vi "AD9959controlAS1_B1.vi"(8 "error in (no error)":errorcluster, 9 "Enable Master Stepper":bool, 10 "Array":T2(array[cluster])=[{"Enable ASF?"=FALSE, "Channel Frequency (MHz)"=80.0, "ASF"=0.12, "Enable Frequency Sweep"=FALSE, "Sweep Parameters"={"Start Frequency (MHz)"=80.5, "Stop Frequency (MHz)"=89.25, "Rising Step Size (MHz)"=0.04375, "Falling Step Size (MHz)"=0.0, "Falling Step Interval (ms)"=0.01, "Rising Step Interval (ms)"=1.0}, "Rising/Falling"=FALSE}, {"Enable ASF?"=TRUE, "Channel Frequency (MHz)"=110.0, "ASF"=0.092, "Enable Frequency Sweep"=TRUE, "Sweep Parameters"={"Start Frequency (MHz)"=70.0, "Stop Frequency (MHz)"=130.0, "Rising Step Size (MHz)"=0.015, "Falling Step Size (MHz)"=0.0, "Falling Step Interval (ms)"=0.01, "Rising Step Interval (ms)"=1.0}, "Rising/Falling"=FALSE}, {"Enable ASF?"=FALSE, "Channel Frequency (MHz)"=80.0, "ASF"=0.1, "Enable Frequency Sweep"=FALSE, "Sweep Parameters"={"Start Frequency (MHz)"=80.5, "Stop Frequency (MHz)"=89.25, "Rising Step Size (MHz)"=0.04375, "Falling Step Size (MHz)"=0.0, "Falling Step Interval (ms)"=0.01, "Rising Step Interval (ms)"=1.0}, "Rising/Falling"=FALSE}, {"Enable ASF?"=TRUE, "Channel Frequency (MHz)"=50.0, "ASF"=0.1, "Enable Frequency Sweep"=FALSE, "Sweep Parameters"={"Start Frequency (MHz)"=40.0, "Stop Frequency (MHz)"=115.0, "Rising Step Size (MHz)"=0.0006, "Falling Step Size (MHz)"=0.0, "Falling Step Interval (ms)"=0.01, "Rising Step Interval (ms)"=1.0}, "Rising/Falling"=FALSE}] {"Sweep Parameters"."Rising Step Interval (ms)" min=0.0 max=2.55 step=0.01 format="%.4f"; "Sweep Parameters"."Stop Frequency (MHz)" min=0.0 max=400.0 step=1.0 format="%.6f"; "Sweep Parameters"."Start Frequency (MHz)" min=0.0 max=400.0 step=1.0 format="%.6f"; "Sweep Parameters"."Falling Step Interval (ms)" min=0.0 max=2.55 step=0.01 format="%.2f"; "Sweep Parameters"."Falling Step Size (MHz)" min=0.0 max=400.0 step=0.1 format="%.6f"; "Sweep Parameters"."Rising Step Size (MHz)" min=0.0 max=400.0 step=0.1 format="%.7f"; "ASF" min=0.0 max=1.0 step=0.001 format="%.3f"; "Channel Frequency (MHz)" min=0.0 max=400.0 step=1.0 format="%.6f"}, 11 "VISA Reference":refnum<visa-resource-name>="AD1") -> (0 "error out":errorcluster, 2 "Duration array":T1(array[cluster])=[{"Number of steps"=4000.0, "Ramp duration (ms)"=4000.0}])   [LabVIEW 2016]
panel:
  out "Actual Channel Frequencies (MHz)":dbl[](array[numeric])=[0.0, 0.0, 0.0, 50.00000001164153] format="%#_10g"
  out "System Clock (MHz)":u32=100
  in  "Multiplier":u32=5
  in  "Reference Clock (MHz)":u32=20
  # "70-130MHz sweep"
  # "40-115MHz sweep"
  # "Notes:\nMinimum Frequency Step is 0.0931 Hz.\nMinimum ASF Step is 0.001"
  # "AD1"
  # "Unused"
  # "AOM3 IntraAction 110 MHz\nProbe 1"
  # "AOM4 Isomet 80 MHz\nCALIBRATION TONE"
  # "AOM3 Intraction 110 MHz\nCalibration tone"
  # "max 0.115"
  # "max 0.185"
  # "max 0.100"
  # "max 0.185"
  # "Channel 1"
  # "Channel 2"
  # "Channel 3"
  # "Channel 0"
  # "I/O"
  # "Clock"
  # "Profile Pins"
  # "P0 is cut\nP1 is cut\nP2 is cut\nP3 is cut"
  # "Power Down"
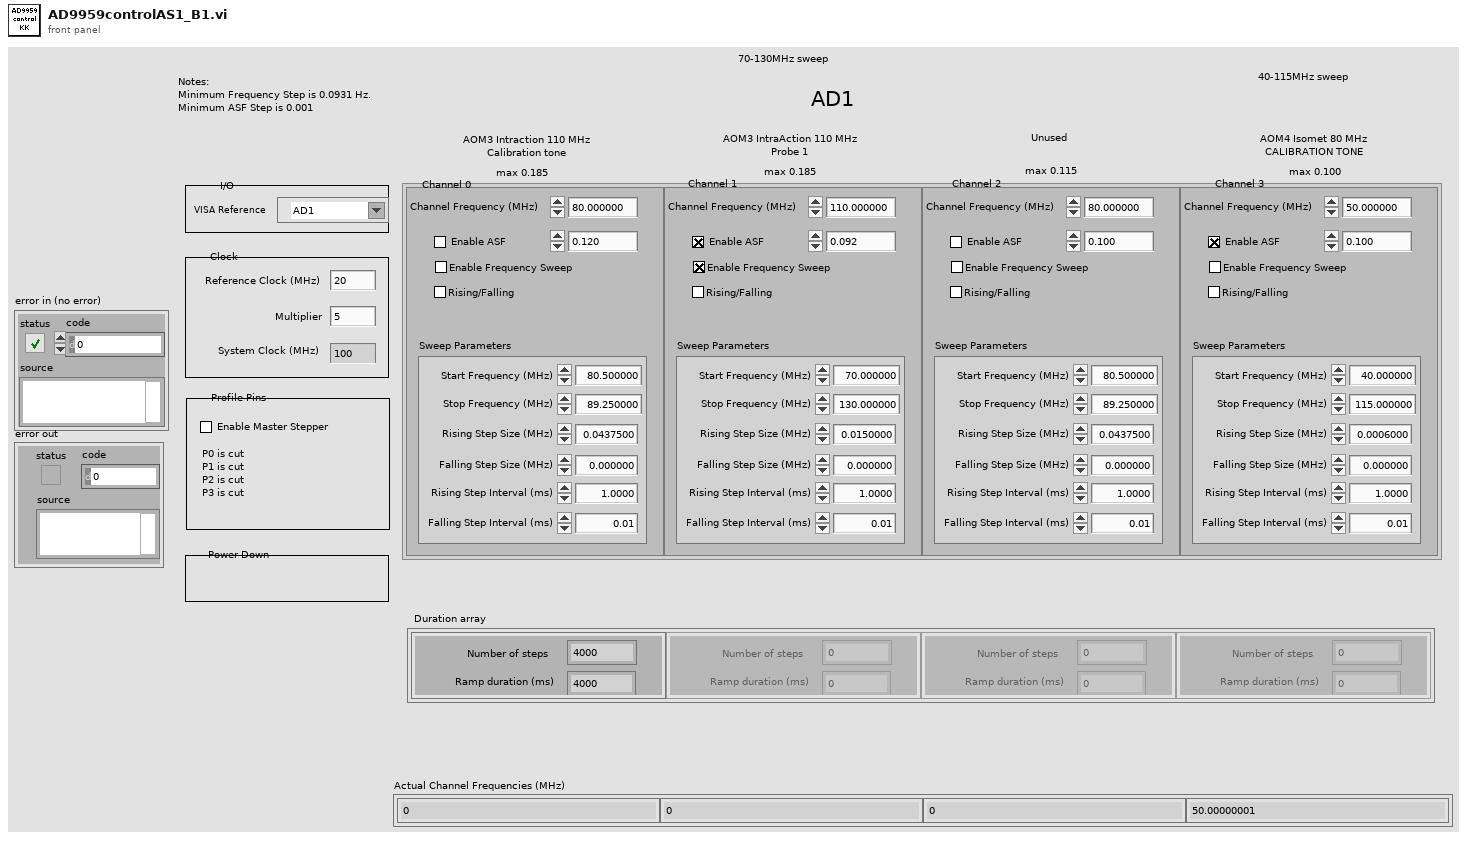
[diagram p1: front panel]
types:
  T1 = cluster{"Number of steps":dbl, "Ramp duration (ms)":dbl}[]
  T2 = cluster{"Enable ASF?":bool, "Channel Frequency (MHz)":dbl, "ASF":dbl, "Enable Frequency Sweep":bool, "Sweep Parameters":cluster{"Start Frequency (MHz)":dbl, "Stop Frequency (MHz)":dbl, "Rising Step Size (MHz)":dbl, "Falling Step Size (MHz)":dbl, "Falling Step Interval (ms)":dbl, "Rising Step Interval (ms)":dbl}, "Rising/Falling":bool}[]
  T3 = cluster{"Start Frequency (MHz)":dbl, "Stop Frequency (MHz)":dbl, "Rising Step Size (MHz)":dbl, "Falling Step Size (MHz)":dbl, "Falling Step Interval (ms)":dbl, "Rising Step Interval (ms)":dbl}[]
  T4 = cluster{"# of steps":dbl, "Ramp duration (ms)":dbl}[]
  T5 = cluster{"# of steps":dbl, "Ramp duration (ms)":dbl}
  T6 = cluster{"Start Frequency (MHz)":dbl, "Stop Frequency (MHz)":dbl, "Rising Step Size (MHz)":dbl, "Falling Step Size (MHz)":dbl, "Falling Step Interval (ms)":dbl, "Rising Step Interval (ms)":dbl}
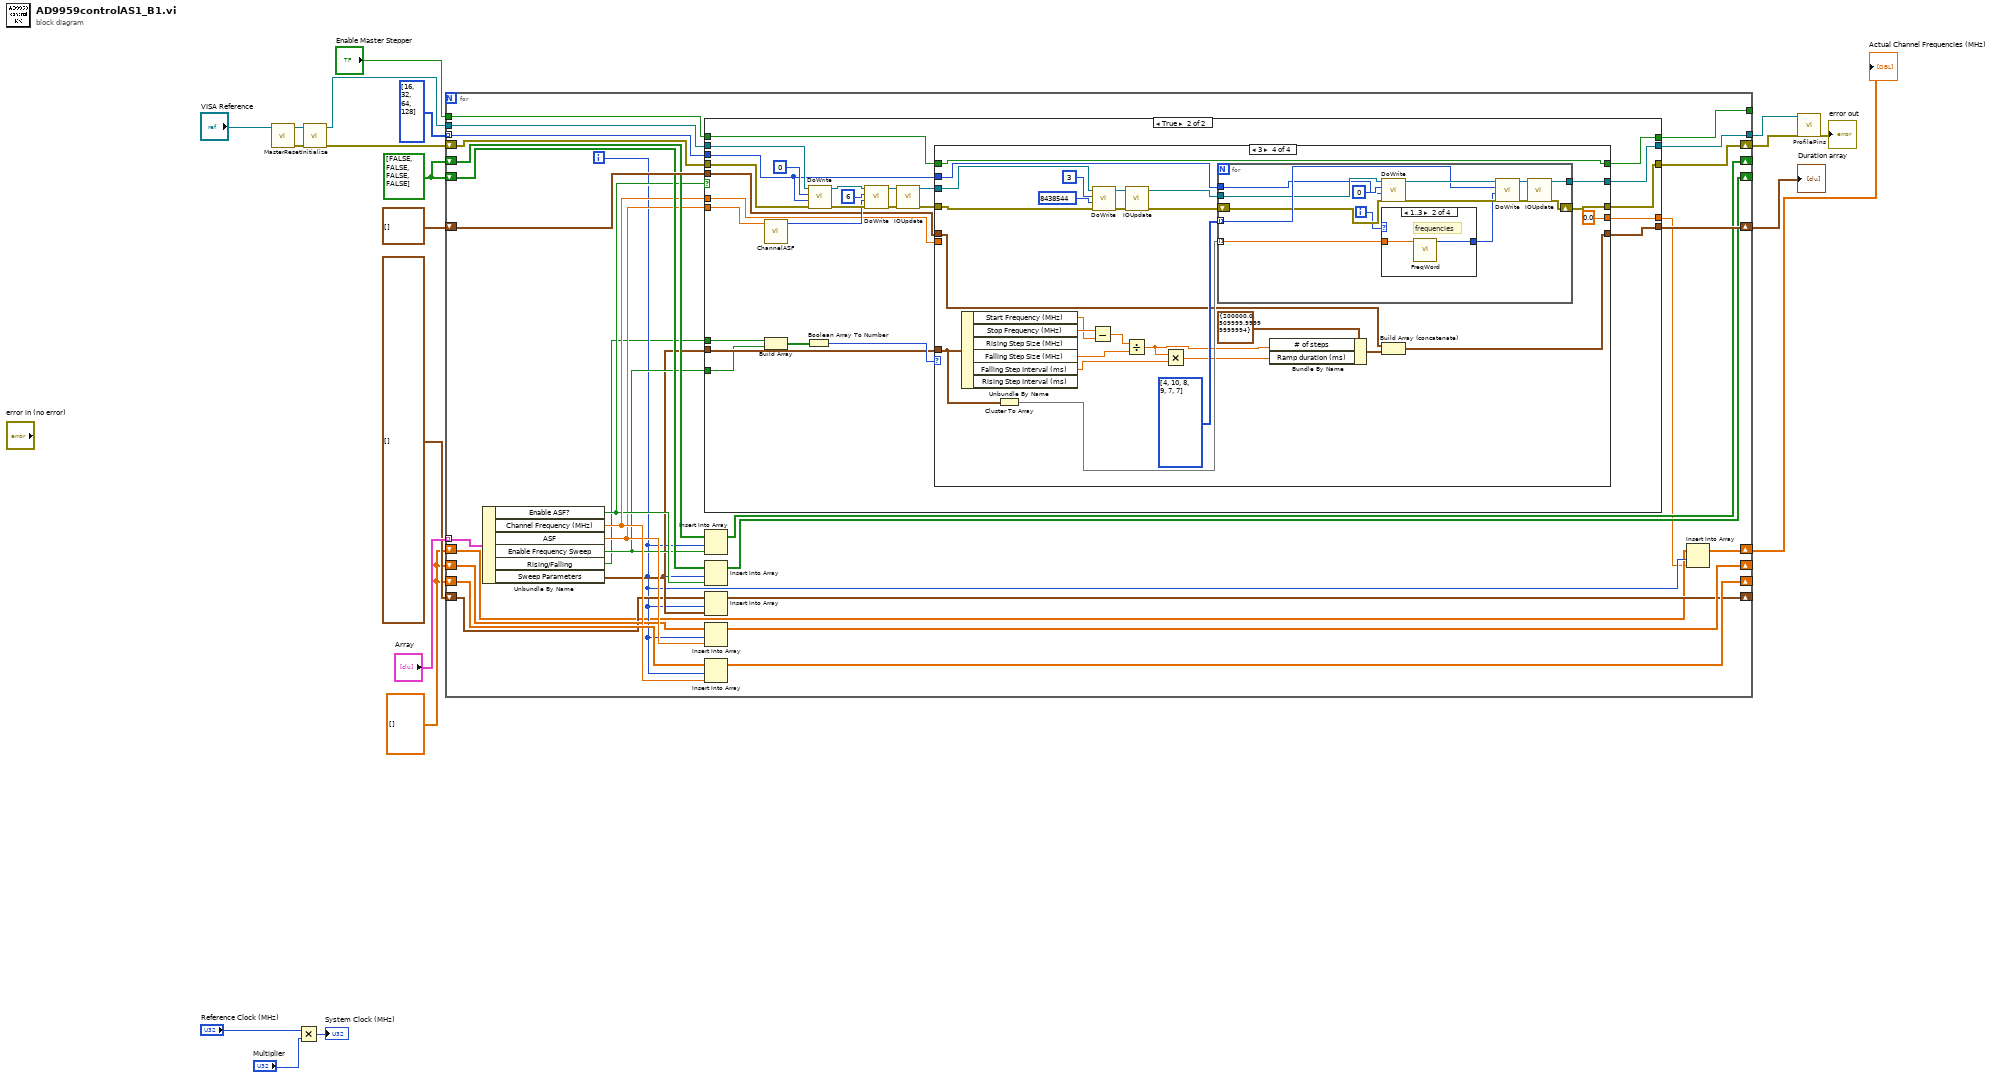
[diagram p0: block diagram]
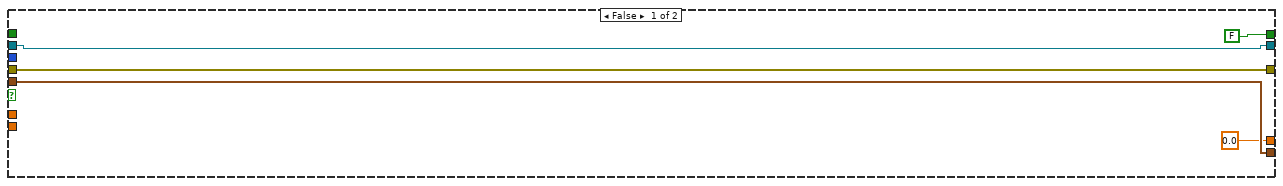
[diagram p2: hidden frame]
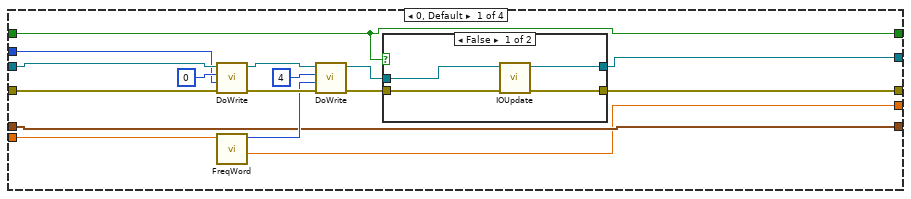
[diagram p3: hidden frame]
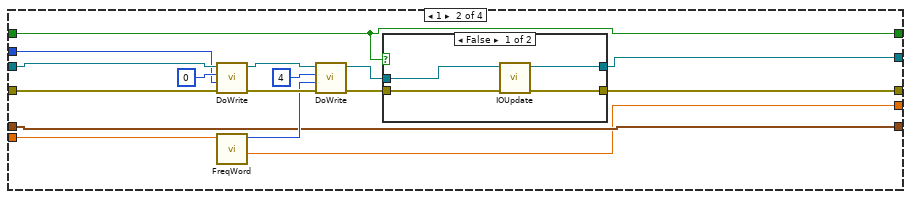
[diagram p5: hidden frame]
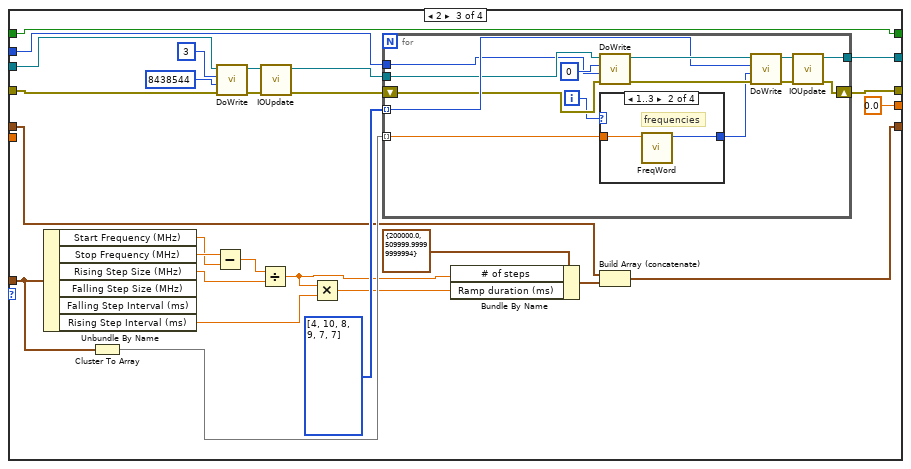
[diagram p7: hidden frame]
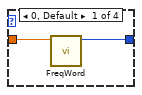
[diagram p8: hidden frame]
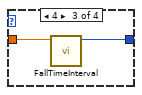
[diagram p9: hidden frame]
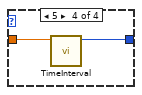
[diagram p10: hidden frame]
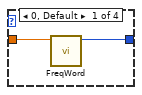
[diagram p11: hidden frame]
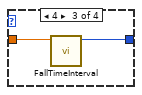
[diagram p12: hidden frame]
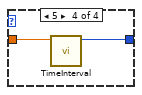
[diagram p13: hidden frame]
diagram:
  w3 = dbl[] [] ("array")
  w8 = bool[] [FALSE, FALSE, FALSE, FALSE] ("element")
  n1 = call "MasterReset.vi"("VISA Reference"="VISA Reference") -> ("error out"=w15:errorcluster, "dup VISA resource name"=w16:refnum<visa-resource-name>)  [unwired: 9 in]
  n2 = Multiply(x="Reference Clock (MHz)", y="Multiplier") -> (x*y=→"System Clock (MHz)":u32)
  n3 = call "Initialize.vi"("error in (no error)"=w15, "VISA Reference"=w16) -> ("error out"=w12:errorcluster, "dup VISA resource name"=w5:refnum<visa-resource-name>)  [unwired: 8 in]
  n4 = for {
    tunnel: "Array" -> [w50] mode=indexing
    tunnel: [w49] -> w4
    tunnel: w5 -> [w48]
    tunnel: u32[] [16, 32, 64, 128] ("Value 3") -> [w46] mode=indexing
    shift-right: [w45] -> w9
    shift-left: T4 [] -> [w44]
    shift-right: [w43] -> w13
    shift-left: w12 -> [w47]
    shift-right: [w41] -> _
    shift-left: w8 -> [w42]
    shift-right: [w39] -> _
    shift-left: w8 -> [w40]
    shift-right: [w36] -> _
    shift-left: w3 -> [w38]
    shift-right: [w32] -> _
    shift-left: w3 -> [w33]
    shift-right: [w28] -> _
    shift-left: T3 [] ("array") -> [w29]
    tunnel: [w27] -> _
    tunnel: "Enable Master Stepper" -> [w26]
    shift-right: [w23] -> w2
    shift-left: w3 -> [w24]
    i -> [w25]
    n5 = Unbundle By Name(w50) -> ("Enable ASF?"=w35:bool, "Channel Frequency (MHz)"=w37:dbl, "ASF"=w34:dbl, "Enable Frequency Sweep"=w31:bool, "Rising/Falling"=w21:bool, "Sweep Parameters"=w30:T6)
    n6 = case shown="True" w35 {
      tunnel: w48 -> [w55 w78]
      tunnel: w47 -> [w54 w79]
      tunnel: [w55 w70] -> w49
      tunnel: [w54 w69] -> w43
      tunnel: w34 -> [_ w68]
      tunnel: w31 -> [_ w57]
      tunnel: w37 -> [_ w67]
      tunnel: w30 -> [_ w59]
      tunnel: w46 -> [_ w66]
      tunnel: [w53 w63] -> w45
      tunnel: w44 -> [w53 w62]
      tunnel: [FALSE ("Enable Master Stepper") w61] -> w27
      tunnel: w26 -> [_ w60]
      tunnel: [0.0 ("Actual Frequency (MHz)") w58] -> w22
      tunnel: w21 -> [_ w56]
      frame False {
      }
      frame True {
        n7 = call "ChannelASF.vi"("ASF"=w68) -> ("ASF in hex"=w72:u32)  [unwired: 10 in]
        n8 = Build Array(w56, w57) -> (w64:bool[])
        n9 = Boolean Array To Number(Boolean array=w64) -> (number=w65:u32)
        n10 = call "DoWrite.vi"("error in (no error)"=w79, "Value"=w66, "Register Address"=0 ("Value 3"), "VISA Reference"=w78) -> ("error out"=w75:errorcluster, "dup VISA resource name"=w77:refnum<visa-resource-name>)  [unwired: 6 in]
        n11 = call "DoWrite.vi"("error in (no error)"=w75, "Value"=w72, "Register Address"=u32 6 ("Register Address 4"), "VISA Reference"=w77) -> ("error out"=w73:errorcluster, "dup VISA resource name"=w76:refnum<visa-resource-name>)  [unwired: 6 in]
        n12 = call "IOUpdate.vi"("error in (no error)"=w73, "VISA Reference"=w76) -> ("error out"=w80:errorcluster, "dup VISA resource name"=w81:refnum<visa-resource-name>)  [unwired: 8 in]
        n13 = case shown="3" w65 {
          tunnel: w80 -> [w90 w112 w149 w198]
          tunnel: w81 -> [w97 w119 w150 w199]
          tunnel: [w88 w110 w142 w191] -> w70
          tunnel: [w87 w109 w141 w190] -> w69
          tunnel: w67 -> [w86 w108 _ _]
          tunnel: w59 -> [_ _ w139 w188]
          tunnel: w66 -> [w85 w107 w140 w189]
          tunnel: [w84 w106 w128 w179] -> w63
          tunnel: w62 -> [w84 w106 w131 w182]
          tunnel: [w83 w105 w127 w178] -> w61
          tunnel: w60 -> [w83 w105 w127 w178]
          tunnel: [w82 w104 0.0 ("Actual Frequency (MHz)") 0.0 ("Actual Frequency (MHz)")] -> w58
          frame 0, Default {
            n14 = call "DoWrite.vi"("error in (no error)"=w90, "Value"=w85, "Register Address"=0 ("Value 3"), "VISA Reference"=w97) -> ("error out"=w96:errorcluster, "dup VISA resource name"=w95:refnum<visa-resource-name>)  [unwired: 6 in]
            n15 = call "FreqWord.vi"("Channel Frequency (MHz)"=w86) -> ("Actual Frequency (MHz)"=w82:dbl, "Frequency Tuning Word"=w91:u32)  [unwired: 9 in]
            n16 = call "DoWrite.vi"("error in (no error)"=w96, "Value"=w91, "Register Address"=u32 4 ("Register Address 2"), "VISA Reference"=w95) -> ("error out"=w93:errorcluster, "dup VISA resource name"=w94:refnum<visa-resource-name>)  [unwired: 6 in]
            n17 = case shown="False" w83 {
              tunnel: w94 -> [w101 w103]
              tunnel: w93 -> [w100 w102]
              tunnel: [w99 w103] -> w88
              tunnel: [w98 w102] -> w87
              frame False {
                n18 = call "IOUpdate.vi"("error in (no error)"=w100, "VISA Reference"=w101) -> ("error out"=w98:errorcluster, "dup VISA resource name"=w99:refnum<visa-resource-name>)  [unwired: 8 in]
              }
              frame True {
              }
            }
          }
          frame 1 {
            n19 = call "DoWrite.vi"("error in (no error)"=w112, "Value"=w107, "Register Address"=0 ("Value 3"), "VISA Reference"=w119) -> ("error out"=w118:errorcluster, "dup VISA resource name"=w117:refnum<visa-resource-name>)  [unwired: 6 in]
            n20 = call "FreqWord.vi"("Channel Frequency (MHz)"=w108) -> ("Actual Frequency (MHz)"=w104:dbl, "Frequency Tuning Word"=w113:u32)  [unwired: 9 in]
            n21 = call "DoWrite.vi"("error in (no error)"=w118, "Value"=w113, "Register Address"=u32 4 ("Register Address 2"), "VISA Reference"=w117) -> ("error out"=w115:errorcluster, "dup VISA resource name"=w116:refnum<visa-resource-name>)  [unwired: 6 in]
            n22 = case shown="False" w105 {
              tunnel: w116 -> [w123 w125]
              tunnel: w115 -> [w122 w124]
              tunnel: [w121 w125] -> w110
              tunnel: [w120 w124] -> w109
              frame False {
                n23 = call "IOUpdate.vi"("error in (no error)"=w122, "VISA Reference"=w123) -> ("error out"=w120:errorcluster, "dup VISA resource name"=w121:refnum<visa-resource-name>)  [unwired: 8 in]
              }
              frame True {
              }
            }
          }
          frame 2 {
            n24 = Unbundle By Name(w139) -> ("Start Frequency (MHz)"=w137:dbl, "Stop Frequency (MHz)"=w138:dbl, "Rising Step Size (MHz)"=w136:dbl, "Rising Step Interval (ms)"=w135:dbl)  [unwired: 2 out]
            n25 = Cluster To Array(cluster=w139) -> (array=w145:dbl[])
            n26 = Subtract(x=w138, y=w137) -> (x-y=w134:dbl)
            n27 = call "DoWrite.vi"("error in (no error)"=w149, "Value"=8438544 ("Value 3"), "Register Address"=3 ("Value 3"), "VISA Reference"=w150) -> ("error out"=w152:errorcluster, "dup VISA resource name"=w151:refnum<visa-resource-name>)  [unwired: 6 in]
            n28 = Divide(x=w134, y=w136) -> (x/y=w130:dbl)
            n29 = call "IOUpdate.vi"("error in (no error)"=w152, "VISA Reference"=w151) -> ("error out"=w144:errorcluster, "dup VISA resource name"=w143:refnum<visa-resource-name>)  [unwired: 8 in]
            n30 = Multiply(x=w130, y=w135) -> (x*y=w129:dbl)
            n31 = for {
              tunnel: i32[] [4, 10, 8, 9, 7, 7] -> [w162] mode=indexing
              shift-right: [w161] -> w141
              shift-left: w144 -> [w160]
              tunnel: w143 -> [w159]
              tunnel: [w154] -> w142
              tunnel: w145 -> [w156] mode=indexing
              tunnel: w140 -> [w153]
              i -> [w157]
              n32 = call "DoWrite.vi"("error in (no error)"=w160, "Value"=w153, "Register Address"=0 ("Value 3"), "VISA Reference"=w159) -> ("error out"=w163:errorcluster, "dup VISA resource name"=w164:refnum<visa-resource-name>)  [unwired: 6 in]
              n33 = case shown="1..3" w157 {
                tunnel: w156 -> [w168 w170 w172 w174]
                tunnel: [w167 w169 w171 w173] -> w155
                frame 0, Default {
                  n34 = call "FreqWord.vi"("Channel Frequency (MHz)"=w168) -> ("Frequency Tuning Word"=w167:u32)  [unwired: 9 in, 1 out]
                }
                frame 1..3 {
                  # "frequencies"
                  n35 = call "FreqWord.vi"("Channel Frequency (MHz)"=w170) -> ("Frequency Tuning Word"=w169:u32)  [unwired: 9 in, 1 out]
                }
                frame 4 {
                  n36 = call "FallTimeInterval.vi"("Fall Time Interval"=w172) -> ("Time interval in Hex"=w171:u32)  [unwired: 10 in]
                }
                frame 5 {
                  n37 = call "TimeInterval.vi"("Time Interval"=w174) -> ("Time interval in Hex"=w173:u32)  [unwired: 10 in]
                }
              }
              n38 = call "DoWrite.vi"("error in (no error)"=w163, "Value"=w155, "Register Address"=w162, "VISA Reference"=w164) -> ("error out"=w165:errorcluster, "dup VISA resource name"=w166:refnum<visa-resource-name>)  [unwired: 6 in]
              n39 = call "IOUpdate.vi"("error in (no error)"=w165, "VISA Reference"=w166) -> ("error out"=w161:errorcluster, "dup VISA resource name"=w154:refnum<visa-resource-name>)  [unwired: 8 in]
            }
            n40 = Bundle By Name(cluster=T5 {"# of steps"=200000.0, "Ramp duration (ms)"=509999.99999999994} ("Duration Cluster"), "# of steps"=w130, "Ramp duration (ms)"=w129) -> (w133:T5)
            n41 = Build Array (concatenate)(w131, w133) -> (w128:T4)
          }
          frame 3 {
            n42 = Unbundle By Name(w188) -> ("Start Frequency (MHz)"=w186:dbl, "Stop Frequency (MHz)"=w187:dbl, "Falling Step Size (MHz)"=w176:dbl, "Falling Step Interval (ms)"=w175:dbl)  [unwired: 2 out]
            n43 = Cluster To Array(cluster=w188) -> (array=w194:dbl[])
            n44 = Subtract(x=w187, y=w186) -> (x-y=w185:dbl)
            n45 = call "DoWrite.vi"("error in (no error)"=w198, "Value"=8438544 ("Value 3"), "Register Address"=3 ("Value 3"), "VISA Reference"=w199) -> ("error out"=w201:errorcluster, "dup VISA resource name"=w200:refnum<visa-resource-name>)  [unwired: 6 in]
            n46 = Divide(x=w185, y=w176) -> (x/y=w181:dbl)
            n47 = call "IOUpdate.vi"("error in (no error)"=w201, "VISA Reference"=w200) -> ("error out"=w193:errorcluster, "dup VISA resource name"=w192:refnum<visa-resource-name>)  [unwired: 8 in]
            n48 = Multiply(x=w181, y=w175) -> (x*y=w180:dbl)
            n49 = for {
              tunnel: i32[] [4, 10, 8, 9, 7, 7] -> [w211] mode=indexing
              shift-right: [w210] -> w190
              shift-left: w193 -> [w209]
              tunnel: w192 -> [w208]
              tunnel: [w203] -> w191
              tunnel: w194 -> [w205] mode=indexing
              tunnel: w189 -> [w202]
              i -> [w206]
              n50 = call "DoWrite.vi"("error in (no error)"=w209, "Value"=w202, "Register Address"=0 ("Value 3"), "VISA Reference"=w208) -> ("error out"=w212:errorcluster, "dup VISA resource name"=w213:refnum<visa-resource-name>)  [unwired: 6 in]
              n51 = case shown="1..3" w206 {
                tunnel: w205 -> [w217 w219 w221 w223]
                tunnel: [w216 w218 w220 w222] -> w204
                frame 0, Default {
                  n52 = call "FreqWord.vi"("Channel Frequency (MHz)"=w217) -> ("Frequency Tuning Word"=w216:u32)  [unwired: 9 in, 1 out]
                }
                frame 1..3 {
                  # "frequencies"
                  n53 = call "FreqWord.vi"("Channel Frequency (MHz)"=w219) -> ("Frequency Tuning Word"=w218:u32)  [unwired: 9 in, 1 out]
                }
                frame 4 {
                  n54 = call "FallTimeInterval.vi"("Fall Time Interval"=w221) -> ("Time interval in Hex"=w220:u32)  [unwired: 10 in]
                }
                frame 5 {
                  n55 = call "TimeInterval.vi"("Time Interval"=w223) -> ("Time interval in Hex"=w222:u32)  [unwired: 10 in]
                }
              }
              n56 = call "DoWrite.vi"("error in (no error)"=w212, "Value"=w204, "Register Address"=w211, "VISA Reference"=w213) -> ("error out"=w214:errorcluster, "dup VISA resource name"=w215:refnum<visa-resource-name>)  [unwired: 6 in]
              n57 = call "IOUpdate.vi"("error in (no error)"=w214, "VISA Reference"=w215) -> ("error out"=w210:errorcluster, "dup VISA resource name"=w203:refnum<visa-resource-name>)  [unwired: 8 in]
            }
            n58 = Bundle By Name(cluster=T5 {"# of steps"=200000.0, "Ramp duration (ms)"=509999.99999999994} ("Duration Cluster"), "# of steps"=w181, "Ramp duration (ms)"=w180) -> (w184:T5)
            n59 = Build Array (concatenate)(w182, w184) -> (w179:T4)
          }
        }
      }
    }
    n60 = Insert Into Array(array=w40, index=w25, new element=w31) -> (w39:bool[])
    n61 = Insert Into Array(array=w42, index=w25, new element=w35) -> (w41:bool[])
    n62 = Insert Into Array(array=w29, index=w25, new element=w30) -> (w28:T3)
    n63 = Insert Into Array(array=w33, index=w25, new element=w34) -> (w32:dbl[])
    n64 = Insert Into Array(array=w38, index=w25, new element=w37) -> (w36:dbl[])
    n65 = Insert Into Array(array=w24, index=w25, new element=w22) -> (w23:dbl[])
  }
  "Duration array" <- w9
  "Actual Channel Frequencies (MHz)" <- w2
  n66 = call "ProfilePins.vi"("error in (no error)"=w13, "VISA Reference"=w4) -> ("error out"=→"error out":errorcluster)  [unwired: 8 in, 1 out]
